vi "GetStateMessage.vi"() -> (3 "GetStateMessage":string)   [LabVIEW 2016]
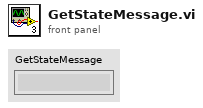
[diagram p1: front panel]
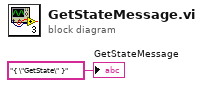
[diagram p0: block diagram]
diagram:
  "GetStateMessage" <- "{ \"GetState\" }" ("GetStateMessage")
